vi "Loop_SEN.vi"() -> ()   [LabVIEW 2017, in "Dashboard.lvlib"]
uses:
  Dashboard.lvlib
  TypeDef/CLUSTER_Limit_Switches.ctl
  _SHARE ALL/Global Share All/Global_STOP.vi
  _SHARE ALL/RoboRio Share All/Systems Share All/Compressor/Globals/GLOBAL_ACT Write_Data_Out.vi
  Globals/Global_CMD_Drive.vi
  WC_Drive/Global_ACT Write_Data Out.vi
  Globals/Global_CMD_Gear.vi
  Globals/Global_Autonomous_Route.vi
  Claw/Global_ACT Write_Data Out.vi
  Lift/Global_ACT Write_Data Out.vi
  Claw Rotation/Global_ACT Write_Data Out.vi
  Arm/Global_ACT Write_Data Out.vi
  Globals/Global_Drive_Turn_sens.vi
  Arm/Global_SM Write_Data Out.vi
  Claw Rotation/Global_SM Write_Data Out.vi
  Lift/Global_SM Write_Data Out.vi
  Globals/Global_Cube_Steering.vi
  _SHARE ALL/RoboRio Share All/Systems Share All/Compressor/Compressor.lvlib
  Global_SEN Write_Data.vi
  VisionHW Folder/VisionHW.lvlib
  Globals/Global_Camera_Ref.vi
  Claw/Claw.lvlib
  Lift/Lift.lvlib
  Claw Rotation/Claw_Rotation.lvlib
  Arm/Arm.lvlib
panel:
  out "Cycle Time (S)":dbl format="%.3g"
  in  "Target Time(ms)":u32=50
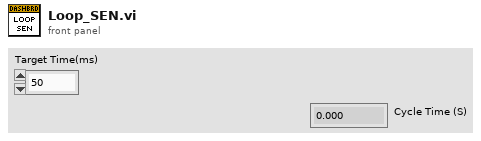
[diagram p1: front panel]
types:
  T1 = cluster{"Target Time(ms)":u32, "Current Time":timestamp, "Previous Time":timestamp, "Cycle Time (S)":dbl, "Num NET Vars":i32}
  T2 = typedef "CLUSTER_Limit_Switches.ctl" = cluster{"Cube":bool, "Top Arm":bool, "Bottom Claw":bool, "Top Lift":bool, "Bottom Arm":bool, "Bottom Lift":bool, "Top Claw":bool}
  T3 = typedef "Cluster_Compressor.ctl" = cluster{"Compressor Running":bool, "Compressor Enabled":bool}
  T4 = typedef "CLUSTER_CMD_WC_Drive.ctl" = cluster{"Drive_Mode":T5, "VBus":T6, "Profile":T8, "Zero Drive Encoders":bool, "Set Target Position(IN)":dbl, "Target Angle(Degree)":dbl, "Lock Angle":bool, "Zero YAW":bool, "Follow Cubes":bool, "Follow Road":bool}
  T5 = typedef "ENUM_WC_Drive_DriveMode.ctl" = enum16{"Motion Profile", "CrossLineAuto", "VBus", "Stop"}
  T6 = typedef "CLUSTER_Drive_ACT Loop_VBus Data.ctl" = cluster{"Drive":T7, "Turbo":bool}
  T7 = typedef "CLUSTER_X and Y.ctl" = cluster{"Steer":dbl, "Throtle":dbl}
  T8 = typedef "CLUSTER_Drive_ACT Loop_Profile Data.ctl" = cluster{"Start":bool}
  T9 = typedef "CLUSTER_Drive_HW_SRX_Status.ctl" = cluster{"Left":T10, "Right":T10}
  T10 = typedef "Cluster_SRX_Common Runtime Data.ctl" = cluster{"Calc":T11, "Voltage ":T12, "Sensor":T13, "Current":dbl, "Temp":dbl}
  T11 = typedef "Cluster_SRX_Error Calculations.ctl" = cluster{"Error":i32, "D-Error":dbl, "I-Acc":dbl}
  T12 = typedef "Cluster_SRX_Voltage Out Data.ctl" = cluster{"Percent":dbl, "Output":dbl, "Bus":dbl}
  T13 = typedef "Cluster_SRX_Sensor Out Data.ctl" = cluster{"Pos":i32, "Vel":i32}
  T14 = typedef "CLUSTER_Drive_Motion Profile Arrays.ctl" = cluster{"Left":T15[], "Right":T15[]}
  T15 = typedef "CLUSTER_Drive_Point Specification.ctl" = cluster{"Position":dbl, "Velocity":dbl, "headingDeg":dbl, "Duration in ms":i32}
  T16 = typedef "WPI_SerialPortRef.ctl" = cluster{"DevStatus":errorcluster, "Serial Port Name":refnum<visa-resource-name>}
  T17 = typedef "ENUM_Auto_AutoMode.ctl" = enum16{"No Movement", "Scale And Switch", "Switch", "Scale", "Cross Line"}
  T18 = typedef "Claw.lvlib/CLUSTER_Limit_Switch_Output.ctl" = cluster{"Limit Switch Output":bool, "Switch Pressed Count":i32}
  T19 = typedef "Lift.lvlib/CLUSTER_ACT_Lift Output.ctl" = cluster{"Common Runtime Data":T10, "Hard Limits":T20}
  T20 = typedef "Cluster_SRX_F and R Limit Indicators.ctl" = cluster{"Forward Closed?":bool, "Reverse Closed?":bool}
  T21 = typedef "Claw_Rotation.lvlib/CLUSTER_ACT_Lift Output.ctl" = cluster{"Common Runtime Data":T10, "Hard Limits":T20}
  T22 = typedef "Arm.lvlib/CLUSTER_ACT_Lift Output.ctl" = cluster{"Common Runtime Data":T10, "Hard Limits":T20}
  T23 = typedef "CLUSTER_Sensitivities.ctl" = cluster{"High Gear Max":dbl, "High Gear Min":dbl, "Low Gear Max":dbl, "Low Gear Min":dbl}
  T24 = typedef "Arm.lvlib/ENUM_SM_State.ctl" = enum16{"Startup", "Idle", "F_Manual", "Manual", "Position - Moving", "Position - Holding", "Shutdown"}
  T25 = typedef "Claw_Rotation.lvlib/ENUM_SM_State.ctl" = enum16{"Startup", "Idle", "F_Manual", "Manual", "Position - Moving", "Position - Holding", "Shutdown"}
  T26 = typedef "Lift.lvlib/ENUM_SM_State.ctl" = enum16{"Startup", "Idle", "F_Manual", "Manual", "Position - Moving", "Position - Holding", "Shutdown"}
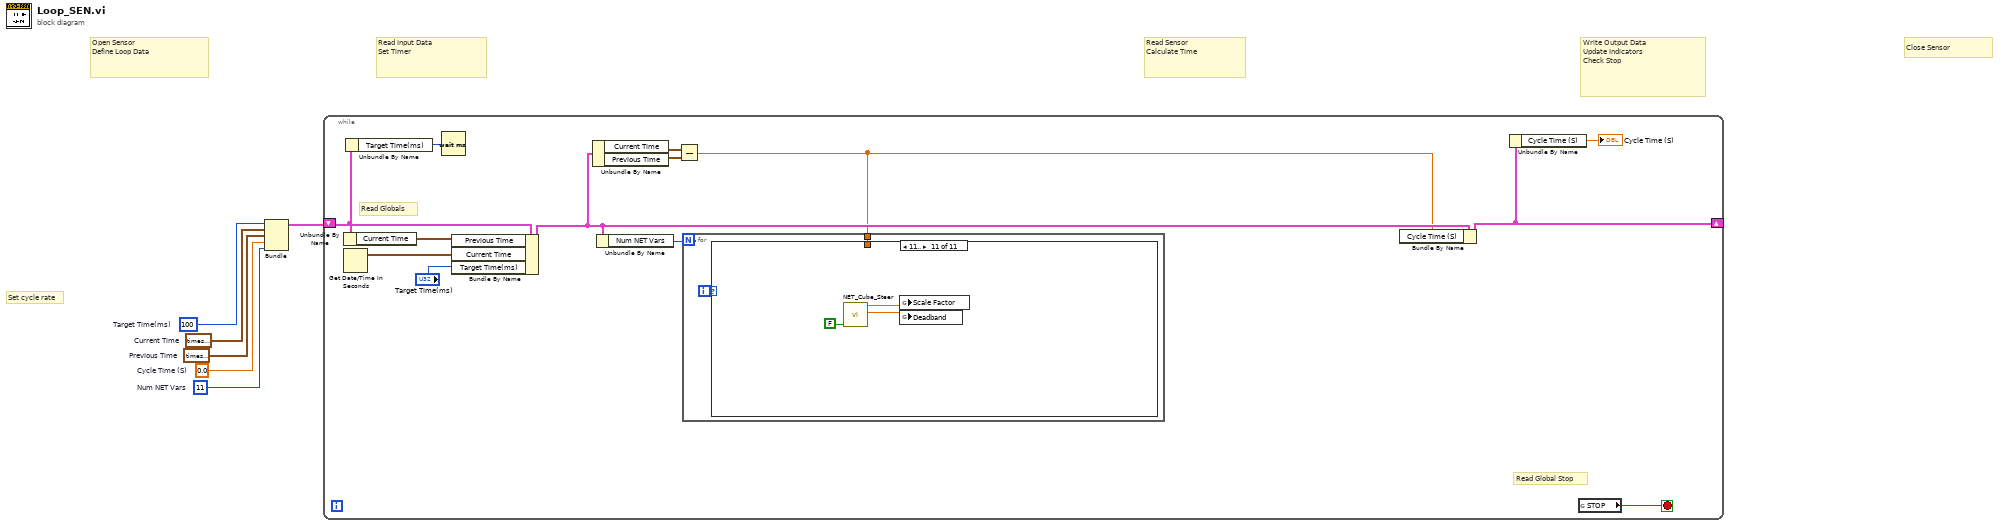
[diagram p0: block diagram]
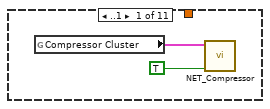
[diagram p2: hidden frame]
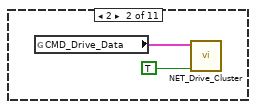
[diagram p3: hidden frame]
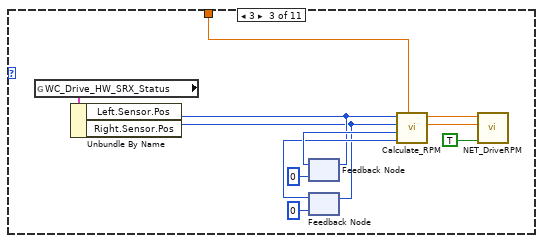
[diagram p4: hidden frame]
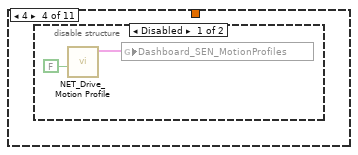
[diagram p5: hidden frame]
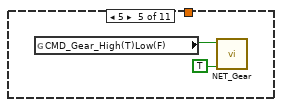
[diagram p7: hidden frame]
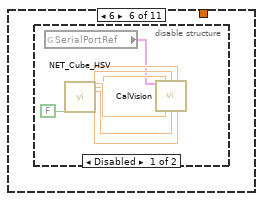
[diagram p8: hidden frame]
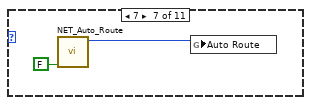
[diagram p10: hidden frame]
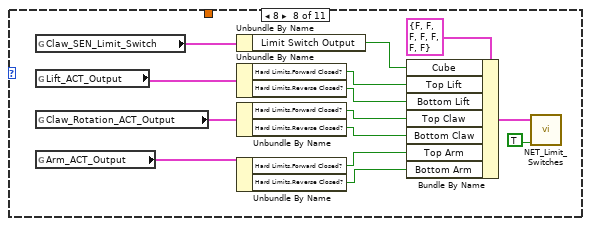
[diagram p11: hidden frame]
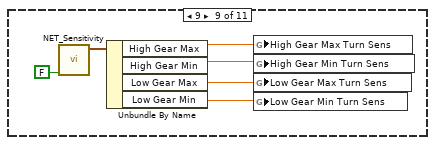
[diagram p12: hidden frame]
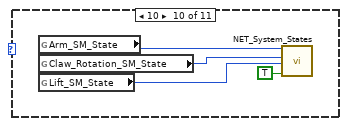
[diagram p13: hidden frame]
diagram:
  w1 = 11  # Num NET Vars
  w2 = 0.0  # Cycle Time (S)
  w6 = timestamp(0 s since 1904-01-01)  # Previous Time
  w5 = timestamp(0 s since 1904-01-01)  # Current Time
  w4 = u32 100  # Target Time(ms)
  # "Close Sensor"
  # "Write Output Data\nUpdate Indicators\nCheck Stop"
  # "Read Sensor\nCalculate Time"
  # "Read Input Data\nSet Timer"
  # "Open Sensor\nDefine Loop Data"
  # "Set cycle rate"
  n1 = Bundle("Target Time(ms)"=w4, "Current Time"=w5, "Previous Time"=w6, "Cycle Time (S)"=w2, "Num NET Vars"=w1) -> (w3:T1)  [unwired: 1 in]
  n2 = while {
    shift-right: [w11] -> _
    shift-left: w3 -> [w13]
    stop <- w19 stop-if-true
    # "Read Globals"
    # "Read Global Stop"
    n3 = Unbundle By Name(w13) -> ("Current Time"=w17:timestamp)
    n4 = Get Date/Time In Seconds() -> (seconds since 1Jan1904=w18:timestamp)
    n5 = Unbundle By Name(w13) -> ("Target Time(ms)"=w12:u32)
    n6 = Wait (ms)(milliseconds to wait=w12) -> ()  [unwired: 1 out]
    n7 = Bundle By Name(cluster=w13, "Previous Time"=w17, "Current Time"=w18, "Target Time(ms)"="Target Time(ms)") -> (w9:T1)
    n8 = Unbundle By Name(w9) -> ("Current Time"=w16:timestamp, "Previous Time"=w15:timestamp)
    n9 = Unbundle By Name(w9) -> ("Num NET Vars"=w8:i32)
    n10 = Subtract(x=w16, y=w15) -> (x-y=w7:dbl)
    n11 = for {
      N: w8 -> [_]
      tunnel: w7 -> [w20]
      i -> [w21]
      n12 = case shown="11.." w21 {
        tunnel: w20 -> [_ _ w35 _ _ _ _ _ _ _ _]
        frame ..1 {
          n13 = global read "GLOBAL_ACT Write_Data_Out.vi" "Compressor Cluster"() -> (w22:T3)
          n14 = call "NET_Compressor.vi"("Read(F) Write(T)"=TRUE, "Compressor  In"=w22) -> ()  [unwired: 9 in, 1 out]
        }
        frame 2 {
          n15 = global read "Global_CMD_Drive.vi" "CMD_Drive_Data"() -> (w24:T4)
          n16 = call "NET_Drive_Cluster.vi"("Read(F) Write(T)"=TRUE, "CMD_DriveCluster"=w24) -> ()  [unwired: 9 in, 1 out]
        }
        frame 3 {
          n17 = global read "Global_ACT Write_Data Out.vi" "WC_Drive_HW_SRX_Status"() -> (w28:T9)
          n18 = Unbundle By Name(w28) -> ("Left.Sensor.Pos"=w27:i32, "Right.Sensor.Pos"=w26:i32)
          n19 = feedback-in #1(w27) -> ()
          n20 = feedback #1(0 ("Numeric")) -> (w32:i32)
          n21 = feedback #2(0 ("Numeric")) -> (w31:i32)
          n22 = feedback-in #2(w26) -> ()
          n23 = call "Calculate_RPM.vi"("ElaspedTime"=w35, "PreviousValueR"=w31, "PreviousValueL"=w32, "CurrentValueR"=w26, "CurrentValueL"=w27) -> ("R RPM OUT"=w29:dbl, "L RPM OUT"=w30:dbl)  [unwired: 5 in]
          n24 = call "NET_DriveRPM.vi"("Read(F) Write(T)"=TRUE, "Right RPM In"=w29, "Left RPM In"=w30) -> ()  [unwired: 7 in, 2 out]
        }
        frame 4 {
          n25 = disable-structure shown="Disabled" {
            frame Disabled {
              n26 = call "NET_Drive_Motion Profile.vi"("Read(F) Write(T)"=FALSE) -> ("Motion Profile Out"=w38:T14)  [unwired: 9 in, 1 out]
              n27 = global write "Global_SEN Write_Data.vi" "Dashboard_SEN_MotionProfiles"(w38) -> ()
            }
            frame Enabled {
            }
          }
        }
        frame 5 {
          n28 = global read "Global_CMD_Gear.vi" "CMD_Gear_High(T)Low(F)"() -> (w39:bool)
          n29 = call "NET_Gear.vi"("Read(F) Write(T)"=TRUE, "High Gear In"=w39) -> ()  [unwired: 9 in, 1 out]
        }
        frame 6 {
          n30 = disable-structure shown="Disabled" {
            frame Disabled {
              n31 = global read "Global_Camera_Ref.vi" "SerialPortRef"() -> (w41:T16)
              n32 = call "NET_Cube_HSV.vi"("Read(F) Write(T)"=FALSE) -> ("H Min Out"=w47:dbl, "H Max Out"=w46:dbl, "S Min Out"=w45:dbl, "S Max Out"=w44:dbl, "V Min Out"=w43:dbl, "V Max Out"=w42:dbl)  [unwired: 21 in]
              n33 = call "CalVision.vi"("SerialPortIn"=w41, "H Max"=w46, "S Max"=w44, "V Max"=w42, "H Min"=w47, "S Min"=w45, "V Min"=w43) -> ()  [unwired: 8 in, 1 out]
            }
            frame Enabled {
            }
          }
        }
        frame 7 {
          n34 = call "NET_Auto_Route.vi"("Read(F) Write(T)"=FALSE) -> ("Route Out"=w50:T17)  [unwired: 10 in]
          n35 = global write "Global_Autonomous_Route.vi" "Auto Route"(w50) -> ()
        }
        frame 8 {
          n36 = global read "Global_ACT Write_Data Out.vi" "Claw_SEN_Limit_Switch"() -> (w61:T18)
          n37 = global read "Global_ACT Write_Data Out.vi" "Lift_ACT_Output"() -> (w63:T19)
          n38 = global read "Global_ACT Write_Data Out.vi" "Claw_Rotation_ACT_Output"() -> (w62:T21)
          n39 = global read "Global_ACT Write_Data Out.vi" "Arm_ACT_Output"() -> (w60:T22)
          n40 = Unbundle By Name(w61) -> ("Limit Switch Output"=w57:bool)
          n41 = Unbundle By Name(w63) -> ("Hard Limits.Forward Closed?"=w56:bool, "Hard Limits.Reverse Closed?"=w55:bool)
          n42 = Unbundle By Name(w62) -> ("Hard Limits.Forward Closed?"=w54:bool, "Hard Limits.Reverse Closed?"=w53:bool)
          n43 = Unbundle By Name(w60) -> ("Hard Limits.Forward Closed?"=w52:bool, "Hard Limits.Reverse Closed?"=w51:bool)
          n44 = Bundle By Name(cluster=T2 {"Cube"=FALSE, "Top Arm"=FALSE, "Bottom Claw"=FALSE, "Top Lift"=FALSE, "Bottom Arm"=FALSE, "Bottom Lift"=FALSE, "Top Claw"=FALSE} ("CLUST_Limit_Switches"), "Cube"=w57, "Top Lift"=w56, "Bottom Lift"=w55, "Top Claw"=w54, "Bottom Claw"=w53, "Top Arm"=w52, "Bottom Arm"=w51) -> (w59:T2)
          n45 = call "NET_Limit_Switches.vi"("Read(F) Write(T)"=TRUE, "Switches In"=w59) -> ()  [unwired: 9 in, 1 out]
        }
        frame 9 {
          n46 = call "NET_Sensitivity.vi"("Read(F) Write(T)"=FALSE) -> ("Sen  Out"=w70:T23)  [unwired: 10 in]
          n47 = Unbundle By Name(w70) -> ("High Gear Max"=w69:dbl, "High Gear Min"=w68:dbl, "Low Gear Max"=w67:dbl, "Low Gear Min"=w66:dbl)
          n48 = global write "Global_Drive_Turn_sens.vi" "High Gear Max Turn Sens"(w69) -> ()
          n49 = global write "Global_Drive_Turn_sens.vi" "High Gear Min Turn Sens"(w68) -> ()
          n50 = global write "Global_Drive_Turn_sens.vi" "Low Gear Max Turn Sens"(w67) -> ()
          n51 = global write "Global_Drive_Turn_sens.vi" "Low Gear Min Turn Sens"(w66) -> ()
        }
        frame 10 {
          n52 = global read "Global_SM Write_Data Out.vi" "Arm_SM_State"() -> (w73:T24)
          n53 = global read "Global_SM Write_Data Out.vi" "Claw_Rotation_SM_State"() -> (w72:T25)
          n54 = global read "Global_SM Write_Data Out.vi" "Lift_SM_State"() -> (w71:T26)
          n55 = call "NET_System_States.vi"("Read(F) Write(T)"=TRUE, "Lift State In"=w71, "Claw Rotation State In"=w72, "Arm State In"=w73) -> ()  [unwired: 5 in, 3 out]
        }
        frame 11.. {
          n56 = call "NET_Cube_Steer.vi"("Read(F) Write(T)"=FALSE) -> ("Deadband Out"=w75:dbl, "Scale Out"=w76:dbl)  [unwired: 9 in]
          n57 = global write "Global_Cube_Steering.vi" "Scale Factor"(w76) -> ()
          n58 = global write "Global_Cube_Steering.vi" "Deadband"(w75) -> ()
        }
      }
    }
    n59 = Bundle By Name(cluster=w9, "Cycle Time (S)"=w7) -> (w11:T1)
    n60 = Unbundle By Name(w11) -> ("Cycle Time (S)"=→"Cycle Time (S)":dbl)
    n61 = global read "Global_STOP.vi" "STOP"() -> (w19:bool)
  }
